vi "Teleop.vi"(10 "Match Info":T1={"Autonomous Elapsed Seconds"=0.0, "TeleOp Elapsed Seconds"=0.0, "Disabled Elapsed Seconds"=0.0, "Visited Autonomous"=FALSE, "Visited TeleOp"=FALSE, "Visited Disabled"=FALSE, "Autonomous Settings"={"Autonomous Style"=enum."Independent", "VI Refnum"=refnum}}, 11 "Call Context":T2) -> ()   [LabVIEW 2017]
doc: "This VI is called for each enabled TeleOp packet received from the DS. It is typically used to read from joysticks and other inputs and update I/O or setpoints for timed control loops. It should complete and return within 20 milliseconds or risk missing DS packets."
uses:
  <vilib>/Rock Robotics/WPI/DriverStation/WPI_DriverStationDerivedRobotMode.ctl
  <vilib>/Rock Robotics/WPI/DriverStation/WPI_DriverStationMatch Info.ctl
  <vilib>/Rock Robotics/WPI/Utilities/WPI_GetSetVariantRefNum.vi
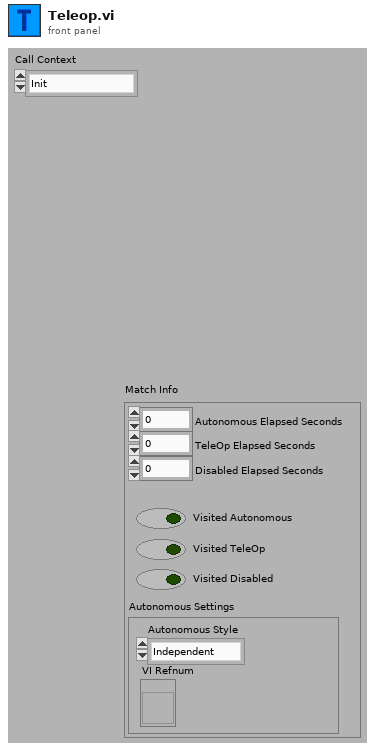
[diagram p1: front panel]
types:
  T1 = typedef "WPI_DriverStationMatch Info.ctl" = cluster{"Autonomous Elapsed Seconds":dbl, "TeleOp Elapsed Seconds":dbl, "Disabled Elapsed Seconds":dbl, "Visited Autonomous":bool, "Visited TeleOp":bool, "Visited Disabled":bool, "Autonomous Settings":cluster{"Autonomous Style":enum16{"Iterative", "Independent"}, "VI Refnum":refnum<vi>}}
  T2 = typedef "WPI_DriverStationDerivedRobotMode.ctl" = enum16{"Init", "Execute", "Stop"}
  T3 = typedef "WPI_JoystickDevRef.ctl" = cluster{"Device":T4}
  T4 = typedef "WPI_JoystickDeviceEnum.ctl" = enum16{"USB 0", "USB 1", "USB 2", "USB 3", "USB 4", "USB 5"}
  T5 = cluster{"Buttons[0]":bool, "Buttons[1]":bool, "Buttons[2]":bool, "Buttons[3]":bool, "Buttons[4]":bool, "Buttons[5]":bool, "Buttons[6]":bool, "Buttons[7]":bool, "Buttons[8]":bool}
  T6 = cluster{"POVs[0]":i16, "POVs[1]":i16, "POVs[2]":i16, "POVs[3]":i16, "POVs[4]":i16, "POVs[5]":i16, "POVs[6]":i16, "POVs[7]":i16, "POVs[8]":i16}
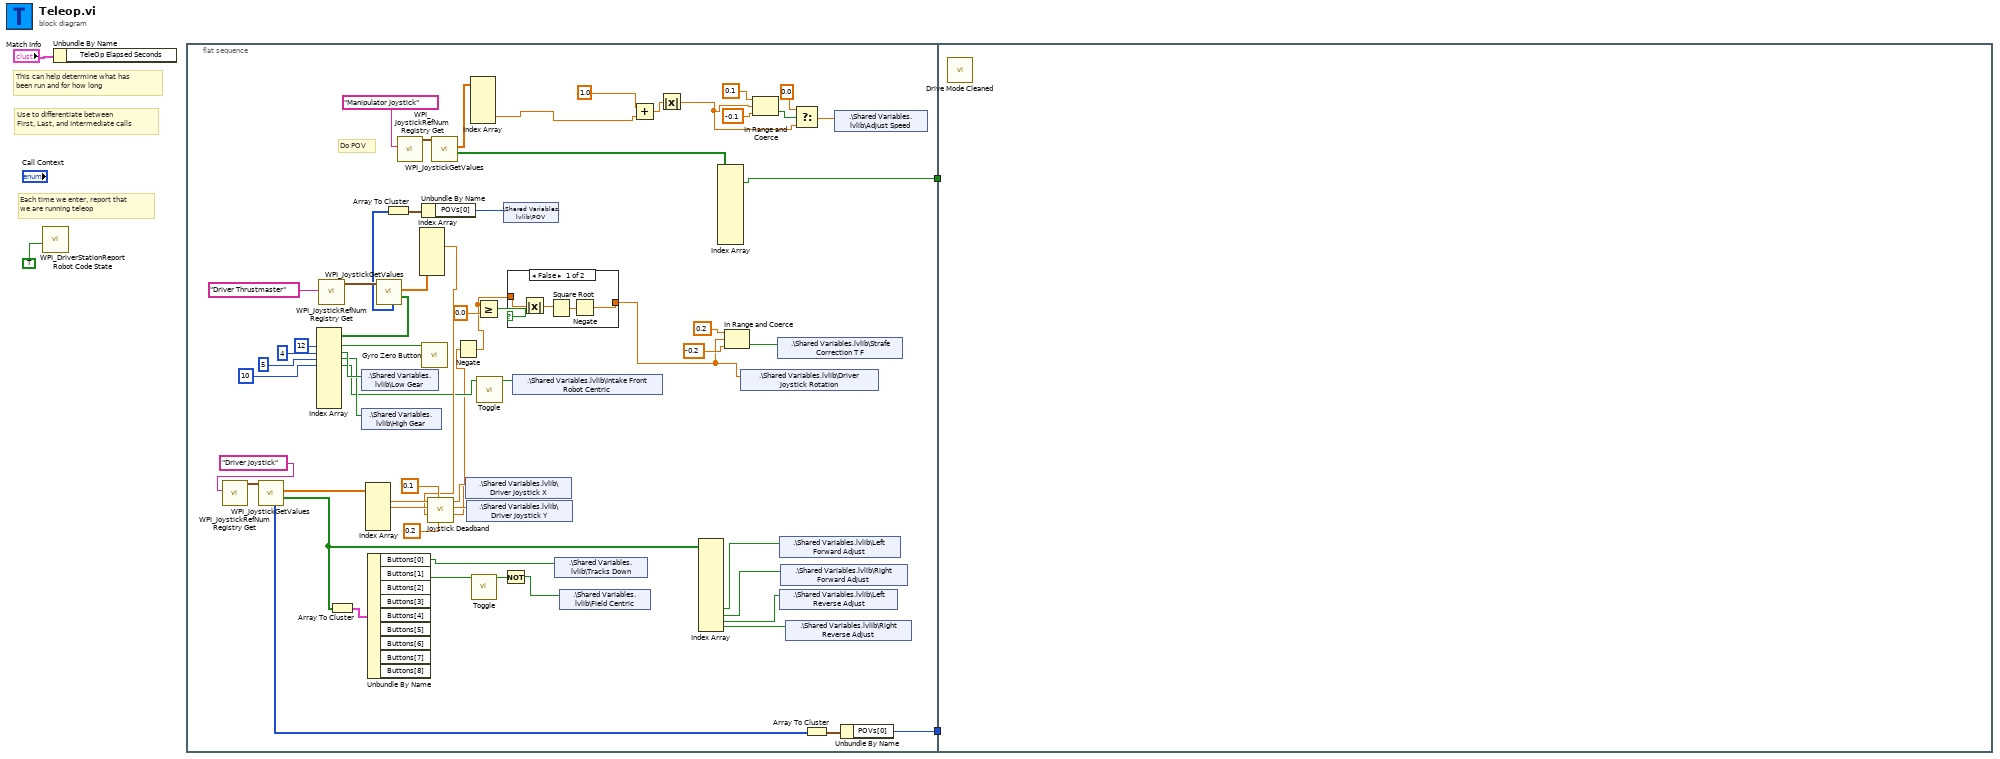
[diagram p0: block diagram]
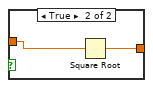
[diagram p2: hidden frame]
diagram:
  # "Each time we enter, report that\nwe are running teleop"
  # "Use to differentiate between\nFirst, Last, and Intermediate calls"
  # "This can help determine what has\nbeen run and for how long"
  n1 = call <vilib>:"WPI_DriverStationReport Robot Code State.vi"("TeleOp"=TRUE ("Autonomous")) -> ()  [unwired: 10 in, 1 out]
  n2 = Unbundle By Name("Match Info") -> ()  [unwired: 1 out]
  n3 = flat-sequence {
    tunnel: [w26] -> w2
    tunnel: [w10] -> w1
    tunnel: w2 -> [_]
    tunnel: w1 -> [_]
    frame #0 {
      # "Do POV"
      n4 = call <vilib>:"WPI_JoystickRefNum Registry Get.vi"("refnum name"="Driver Joystick") -> ("JoystickDevRef"=w65:T3)  [unwired: 1 in, 9 out]
      n5 = call <vilib>:"WPI_JoystickGetValues.vi"("JoystickDevRef"=w65) -> ("Buttons"=w36:bool[], "Axes"=w63:dbl[], "POVs"=w11:i16[])  [unwired: 6 in, 2 out]
      n6 = call <vilib>:"WPI_JoystickRefNum Registry Get.vi"("refnum name"="Driver Thrustmaster") -> ("JoystickDevRef"=w46:T3)  [unwired: 9 in, 1 out]
      n7 = Array To Cluster(array=w36) -> (cluster=w62:T5)
      n8 = Index Array(array=w63) -> (element #1=w53:dbl, element #2=w52:dbl)  [unwired: 5 in, 3 out]
      n9 = Unbundle By Name(w62) -> ("Buttons[0]"=w50:bool, "Buttons[1]"=w54:bool)  [unwired: 7 out]
      n10 = call <vilib>:"WPI_JoystickGetValues.vi"("JoystickDevRef"=w46) -> ("Buttons"=w25:bool[], "Axes"=w45:dbl[], "POVs"=w13:i16[])  [unwired: 6 in, 2 out]
      n11 = Index Array(array=w25, index #1=12 ("index"), index #2=4 ("index"), index #3=5 ("index"), index #4=10 ("index")) -> (element #1=w23:bool, element #2=w20:bool, element #3=w19:bool, element #4=w14:bool)  [unwired: 6 in, 6 out]
      n12 = shared-variable ".\\Shared Variables.lvlib\\Low Gear"(w20) -> ()  [unwired: 1 in, 1 out]
      n13 = shared-variable ".\\Shared Variables.lvlib\\High Gear"(w19) -> ()  [unwired: 1 in, 1 out]
      n14 = Array To Cluster(array=w13) -> (cluster=w18:T6)
      n15 = call <vilib>:"WPI_JoystickRefNum Registry Get.vi"("refnum name"="Manipulator Joystick") -> ("JoystickDevRef"=w60:T3)  [unwired: 1 in, 9 out]
      n16 = Index Array(array=w45) -> (element #1=w29:dbl)  [unwired: 5 in, 4 out]
      n17 = Unbundle By Name(w18) -> ("POVs[0]"=w17:i16)
      n18 = call "Gyro Zero Button.vi"("Boolean"=w23) -> ()  [unwired: 11 in]
      n19 = call "Joystick Deadband.vi"("Z Deadband"=0.2, "X Y Deadband"=0.1, "Z"=w29, "Y"=w52, "X"=w53) -> ("Z Out"=w7:dbl, "Y Out"=w57:dbl, "X Out"=w58:dbl)  [unwired: 4 in]
      n20 = call <vilib>:"WPI_JoystickGetValues.vi"("JoystickDevRef"=w60) -> ("Buttons"=w55:bool[], "Axes"=w41:dbl[])  [unwired: 6 in, 3 out]
      n21 = Negate(x=w7) -> (-x=w8:dbl)
      n22 = shared-variable ".\\Shared Variables.lvlib\\Driver Joystick X"(w58) -> ()  [unwired: 1 in, 1 out]
      n23 = shared-variable ".\\Shared Variables.lvlib\\Driver Joystick Y"(w57) -> ()  [unwired: 1 in, 1 out]
      n24 = Index Array(array=w41) -> (element #3=w32:dbl)  [unwired: 5 in, 4 out]
      n25 = call "Toggle.vi"("Input"=w54) -> ("Output"=w56:bool)  [unwired: 9 in, 1 out]
      n26 = Greater Or Equal?(x=w8, y=0.0) -> (x >= y?=w31:bool)
      n27 = call "Toggle.vi"("Input"=w14) -> ("Output"=w15:bool)  [unwired: 9 in, 1 out]
      n28 = shared-variable ".\\Shared Variables.lvlib\\POV"(w17) -> ()  [unwired: 1 in, 1 out]
      n29 = Not(x=w56) -> (.not. x?=w51:bool)
      n30 = case shown="False" w31 {
        tunnel: [w67 w71] -> w28
        tunnel: w8 -> [w66 w70]
        frame False {
          n31 = Absolute Value(x=w66) -> (abs(x)=w69:dbl)
          n32 = Square Root(x=w69) -> (sqrt(x)=w68:dbl)
          n33 = Negate(x=w68) -> (-x=w67:dbl)
        }
        frame True {
          n34 = Square Root(x=w70) -> (sqrt(x)=w71:dbl)
        }
      }
      n35 = shared-variable ".\\Shared Variables.lvlib\\Intake Front Robot Centric"(w15) -> ()  [unwired: 1 in, 1 out]
      n36 = shared-variable ".\\Shared Variables.lvlib\\Tracks Down"(w50) -> ()  [unwired: 1 in, 1 out]
      n37 = shared-variable ".\\Shared Variables.lvlib\\Field Centric"(w51) -> ()  [unwired: 1 in, 1 out]
      n38 = Add(x=1.0, y=w32) -> (x+y=w35:dbl)
      n39 = Absolute Value(x=w35) -> (abs(x)=w33:dbl)
      n40 = Index Array(array=w36) -> (element #9=w49:bool, element #10=w48:bool, element #11=w6:bool, element #12=w5:bool)  [unwired: 12 in, 8 out]
      n41 = Index Array(array=w55) -> (element #1=w26:bool)  [unwired: 10 in, 9 out]
      n42 = In Range and Coerce(upper limit=0.2, x=w28, lower limit=-0.2) -> (In Range?=w44:bool)  [unwired: 1 out]
      n43 = shared-variable ".\\Shared Variables.lvlib\\Driver Joystick Rotation"(w28) -> ()  [unwired: 1 in, 1 out]
      n44 = In Range and Coerce(upper limit=0.1, x=w33, lower limit=-0.1 ("x")) -> (In Range?=w38:bool)  [unwired: 1 out]
      n45 = shared-variable ".\\Shared Variables.lvlib\\Strafe Correction T F"(w44) -> ()  [unwired: 1 in, 1 out]
      n46 = shared-variable ".\\Shared Variables.lvlib\\Left Forward Adjust"(w49) -> ()  [unwired: 1 in, 1 out]
      n47 = shared-variable ".\\Shared Variables.lvlib\\Left Reverse Adjust"(w6) -> ()  [unwired: 1 in, 1 out]
      n48 = shared-variable ".\\Shared Variables.lvlib\\Right Forward Adjust"(w48) -> ()  [unwired: 1 in, 1 out]
      n49 = shared-variable ".\\Shared Variables.lvlib\\Right Reverse Adjust"(w5) -> ()  [unwired: 1 in, 1 out]
      n50 = Select(t=0.0, s=w38, f=w33) -> (s? t:f=w27:dbl)
      n51 = Array To Cluster(array=w11) -> (cluster=w12:T6)
      n52 = shared-variable ".\\Shared Variables.lvlib\\Adjust Speed"(w27) -> ()  [unwired: 1 in, 1 out]
      n53 = Unbundle By Name(w12) -> ("POVs[0]"=w10:i16)
    }
    frame #1 {
      n54 = call "Drive Mode Cleaned.vi"() -> ()  [unwired: 12 in]
    }
  }
